vi "ReadABF1x.vi"(8 "error in (no error)":errorcluster caption="에러 입력(에러 없음)", 10 "FilePath":path=path "C:/Users/KimYG/Experimental Data/Flocculus_Ex vivo/6. Plsticity/190119/190119_#07/190119__0026.abf", 11 "ABF1FIO 입력":refnum<class "ABF1FIO.lvclass">) -> (0 "error out":errorcluster caption="에러 출력", 3 "ABF1FIO 출력":refnum<class "ABF1FIO.lvclass">)   [LabVIEW 2017, in "ABF1FIO.lvclass"]
uses:
  ABF1FIO.lvclass
  ABF1FIO.lvclass/ABF1FIO.ctl
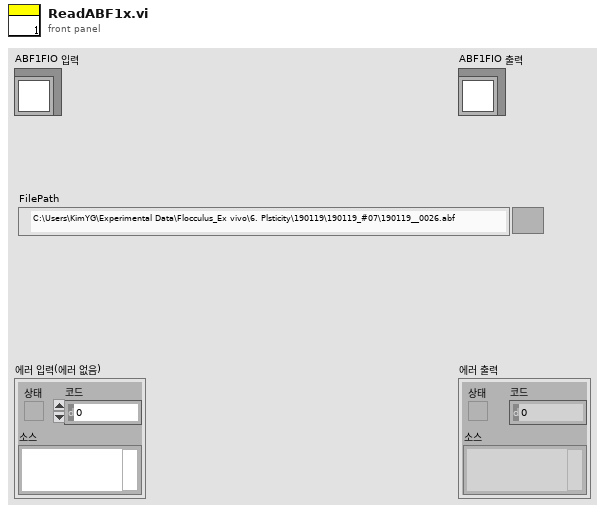
[diagram p1: front panel]
types:
  T1 = enum16{"big-endian, network order", "native, host order", "little-endian"}
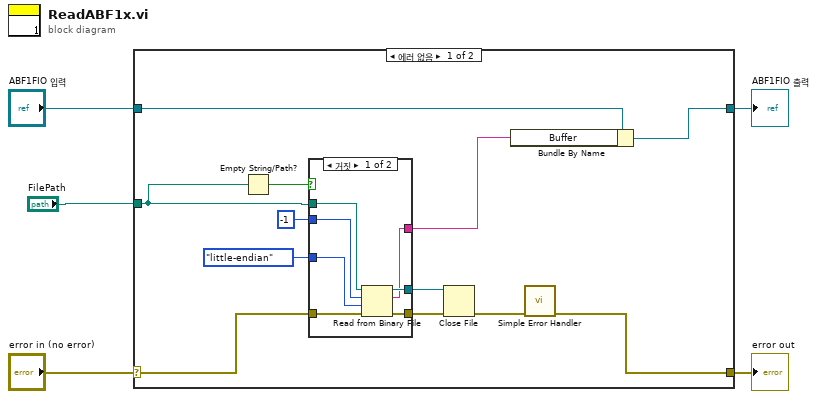
[diagram p0: block diagram]
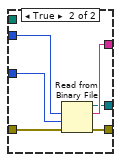
[diagram p2: hidden frame]
diagram:
  n1 = case shown="에러 없음" "error in (no error)" {
    selector: "error in (no error)" -> [w10 w32]
    tunnel: [w9 w32] -> w4
    tunnel: [w7 w31] -> w2
    tunnel: "ABF1FIO 입력" -> [w8 w31]
    tunnel: "FilePath" -> [w6 _]
    frame No Error {
      n2 = Empty String/Path?(string/path=w6) -> (empty?=w15:bool)
      n3 = case shown="거짓" w15 {
        tunnel: T1."little-endian" ("바이트 순서(0:big-endian, network order)") -> [w24 w28]
        tunnel: [w23 w25] -> w17
        tunnel: [w22 w29] -> w12
        tunnel: w10 -> [w21 w30]
        tunnel: -1 ("numBytes") -> [w20 w27]
        tunnel: [w19 w26] -> w16
        tunnel: w6 -> [w18 _]
        frame False {
          n4 = Read from Binary File(8:w21, 9:w24, 10:w20, 11:w18) -> (0:w22:errorcluster, 2:w19:string, 3:w23:refnum<file>)  [unwired: 2 in, 1 out]
        }
        frame True {
          n5 = Read from Binary File(8:w30, 9:w28, 10:w27) -> (0:w29:errorcluster, 2:w26:string, 3:w25:refnum<file>)  [unwired: 3 in, 1 out]
        }
      }
      n6 = Close File(refnum=w17, error in=w12) -> (error out=w13:errorcluster)  [unwired: 1 out]
      n7 = Bundle By Name(cluster=w8, "Buffer"=w16) -> (w7:refnum<class "ABF1FIO.lvclass">)
      n8 = call <vilib>:"Simple Error Handler.vi"("error in (no error)"=w13) -> ("error out"=w9:errorcluster)  [unwired: 4 in, 4 out]
    }
    frame Error {
    }
  }
  "error out" <- w4
  "ABF1FIO 출력" <- w2
